vi "Create All Message Queues_myRio.vi"(8 "error in (no error)":errorcluster) -> (0 "error out":errorcluster, 3 "Queues":T1)   [LabVIEW 2015]
doc: "This VI creates and initializes all the message queues for your application. If your application requires more than one message queue, right-click the \"Message Queues\" constant above and select Open Type Def. Add the new Message Queue(s) to the type definition, then initialize them in this VI."
uses:
  Queues.ctl
  Program Files/National Instruments/LabVIEW 2015/ProjectTemplates/Source/Core/Queued Message Handler/support/Message Queue/Message Cluster.ctl
  Program Files/National Instruments/LabVIEW 2015/ProjectTemplates/Source/Core/Queued Message Handler/support/Message Queue/Enqueue Message (Single).vi
  Program Files/National Instruments/LabVIEW 2015/ProjectTemplates/Source/Core/Queued Message Handler/support/Message Queue/Message Queue.lvlib
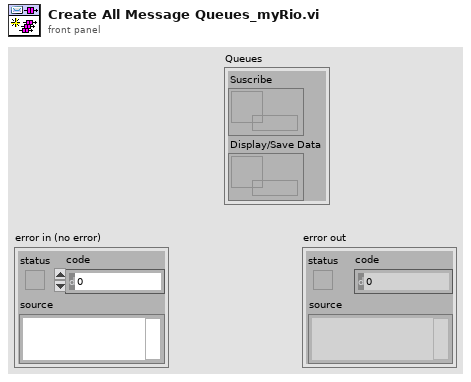
[diagram p1: front panel]
types:
  T1 = typedef "Queues.ctl" = cluster{"Suscribe":refnum<queue>, "Display/Save Data":refnum<queue>}
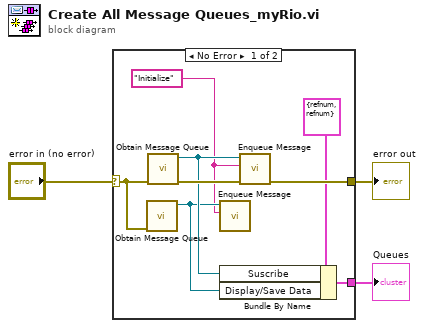
[diagram p0: block diagram]
diagram:
  n1 = case shown="No Error" "error in (no error)" {
    selector: "error in (no error)" -> [w6 w12]
    tunnel: [w11 w12] -> w3
    tunnel: [w10 _] -> w1
    frame No Error {
      w4 = "Initialize" ("Message")
      n2 = call "Obtain Message Queue.vi"("error in (no error)"=w6) -> ("Message Queue"=w5:refnum<queue>)  [unwired: 9 in, 1 out]
      n3 = call "Obtain Message Queue.vi"("error in (no error)"=w6) -> ("error out"=w9:errorcluster, "Message Queue"=w8:refnum<queue>)  [unwired: 9 in]
      n4 = call-poly "Enqueue Message.vi"("Message"=w4, "Message Queue"=w5) -> ()  [unwired: 8 in, 2 out]
      n5 = Bundle By Name(cluster=T1 {"Suscribe"=refnum, "Display/Save Data"=refnum}, "Suscribe"=w8, "Display/Save Data"=w5) -> (w10:T1)
      n6 = call-poly "Enqueue Message.vi"("error in (no error)"=w9, "Message"=w4, "Message Queue"=w8) -> ("error out"=w11:errorcluster)  [unwired: 7 in, 1 out]
    }
    frame Error {
    }
  }
  "error out" <- w3
  "Queues" <- w1
